vi "SetConfig(SubVI).vi"(0 "Name 3":string, 5 "Array Oy 2":string, 7 "Array Ox 2":string, 9 "Line Width 2":string, 11 "Line Color 4":string(combo)) -> ()   [LabVIEW 2018]
panel:
  out "Entered username":string
  out "Entered password":string
  in  "Enter Username":string
  in  "Enter Password":string
  out "Cancelled?":bool
  in  "Line Color 3":string
  in  "Ok":bool
  in  "Name 2":string
  in  "Line Color 2":string(combo)
  in  "Line Color":string
  in  "Array Oy":string
  in  "Array Ox":string
  in  "Line Width":string
  # "Line"
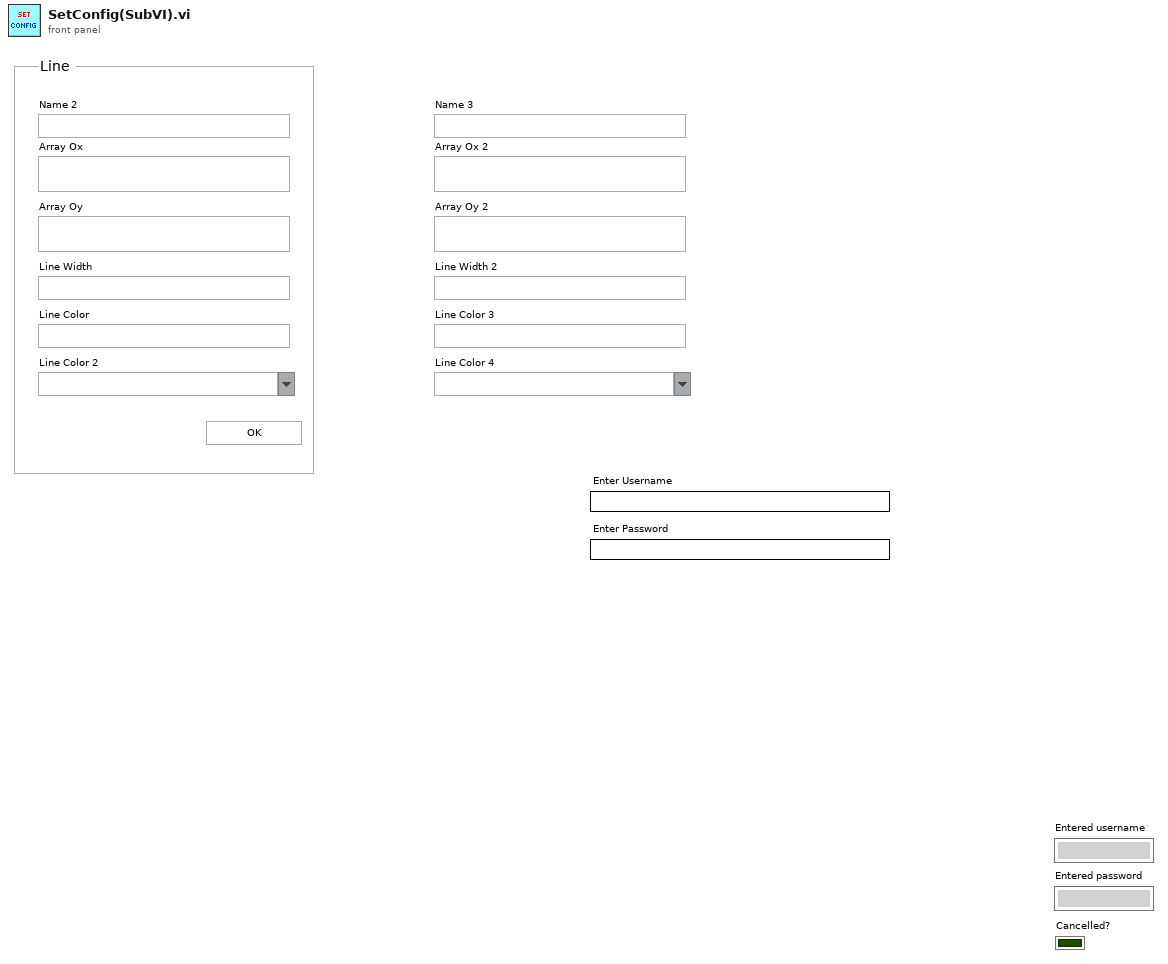
[diagram p1: front panel]
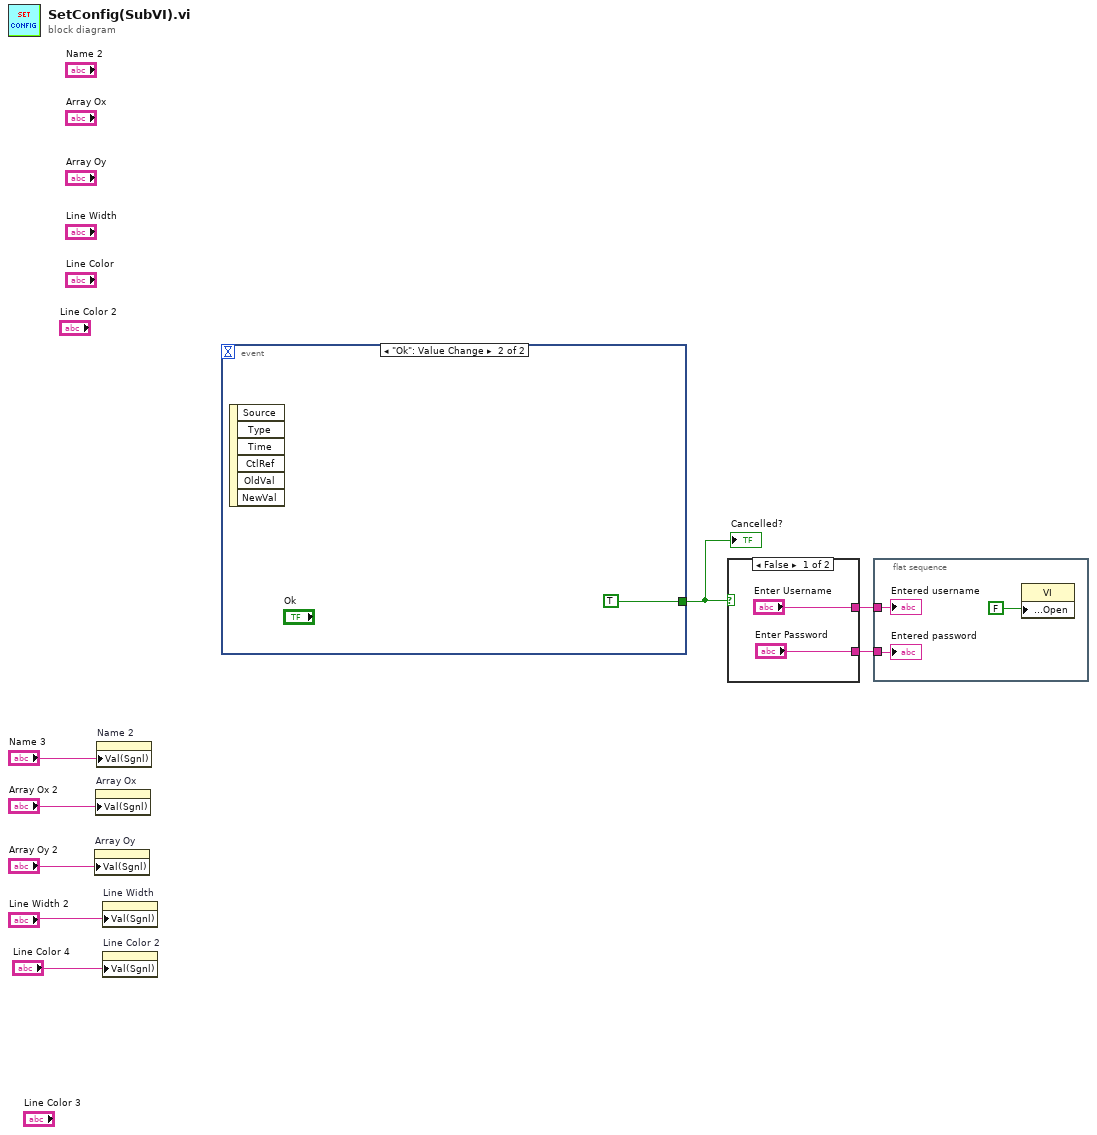
[diagram p0: block diagram]
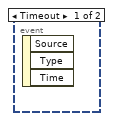
[diagram p3: hidden frame]
diagram:
  n1 = property on="Array Oy" class="Str"("Val(Sgnl)"="Array Oy 2") -> ()  [unwired: 2 in, 2 out]
  n2 = property on="Array Ox" class="Str"("Val(Sgnl)"="Array Ox 2") -> ()  [unwired: 2 in, 2 out]
  n3 = property on="Name 2" class="Str"("Val(Sgnl)"="Name 3") -> ()  [unwired: 2 in, 2 out]
  n4 = property on="Line Width" class="Str"("Val(Sgnl)"="Line Width 2") -> ()  [unwired: 2 in, 2 out]
  n5 = property on="Line Color 2" class="CmbBox"("Val(Sgnl)"="Line Color 4") -> ()  [unwired: 2 in, 2 out]
  n6 = event shown="[1] \"Ok\": Value Change" {
    selector: _ -> [_ _]
    dyn-events: _ -> [_ _]
    timeout: _ -> [_ _]
    tunnel: [_ TRUE] -> w1
    event Timeout {
      n7 = event-data() -> ()  [unwired: 1 in, 3 out]
    }
    event "Ok": Value Change {
      n8 = event-data() -> ()  [unwired: 1 in, 6 out]
    }
  }
  "Cancelled?" <- w1
  n9 = case shown="False" w1 {
    tunnel: ["Enter Username" _] -> w3
    tunnel: ["Enter Password" _] -> w2
    frame False {
    }
    frame True {
    }
  }
  n10 = flat-sequence {
    tunnel: w3 -> [w13]
    tunnel: w2 -> [w12]
    frame #0 {
      n11 = property class="VI"("Front Panel.Open"=FALSE ("Front Panel Window:Open")) -> ()  [unwired: 2 in, 2 out]
      "Entered username" <- w13
      "Entered password" <- w12
    }
  }
